vi "svfa_Check Data Valid [Dual FFT].vi"(0 "stimulus [X]":waveform(dbl)={"t0"=timestamp(0 s since 1904-01-01), "dt"=1.953125e-05, "Y"=[]}, 1 "response [Y]":waveform(dbl)={"t0"=timestamp(0 s since 1904-01-01), "dt"=1.953125e-05, "Y"=[]}, 2 "window":T3=1 items=["None"=0, "Hanning"=1, "Hamming"=2, "Blackman-Harris"=3, "Exact Blackman"=4, "Blackman"=5, "Flat Top"=6, "4 Term B-Harris "=7, "7 Term B-Harris"=8, "Low Sidelobe"=9, "Force - Exponential"=10, "Blackman Nuttall"=11, "Triangle"=30, "Bartlett-Hanning"=31, "Bohman"=32, "Parzen"=33, "Welch"=34, "Kaiser"=60, "Dolph-Chebyshev"=61, "Gaussian"=62], 3 "force/exp settings":T2={"force window [%]"=50.0, "exp window [%]"=10.0} {"exp window [%]" min=0.0 max=100.0 format="%.2f"; "force window [%]" min=0.0 max=100.0 format="%.2f"}, 4 "averaging parameters":T5={"averaging mode"=enum."No averaging", "weighting mode"=enum."Linear", "number of averages"=10, "linear mode"=enum."Auto restart"}, 5 "error in (no error)":errorcluster, 7 "processing control in":T4(ring), 8 "restart averaging (F)":bool, 9 "FRF mode":enum16{"H1", "H2", "H3"}(ring), 10 "measurement":T1(ring)=enum."Frequency response") -> (11 "dup FRF mode":enum16{"H1", "H2", "H3"}(ring), 13 "processing control out":T4(ring), 14 "dup stimulus [X]":waveform(dbl)={"t0"=timestamp(0 s since 1904-01-01), "dt"=1.953125e-05, "Y"=[]}, 15 "dup response [Y]":waveform(dbl)={"t0"=timestamp(0 s since 1904-01-01), "dt"=1.953125e-05, "Y"=[]}, 16 "window":T3=1 items=["None"=0, "Hanning"=1, "Hamming"=2, "Blackman-Harris"=3, "Exact Blackman"=4, "Blackman"=5, "Flat Top"=6, "4 Term B-Harris "=7, "7 Term B-Harris"=8, "Low Sidelobe"=9, "Force - Exponential"=10, "Blackman Nuttall"=11, "Triangle"=30, "Bartlett-Hanning"=31, "Bohman"=32, "Parzen"=33, "Welch"=34, "Kaiser"=60, "Dolph-Chebyshev"=61, "Gaussian"=62], 17 "dup force/exp settings":T2={"force window [%]"=50.0, "exp window [%]"=10.0} {"exp window [%]" min=0.0 max=100.0 format="%.2f"; "force window [%]" min=0.0 max=100.0 format="%.2f"}, 18 "dup averaging parameters":T5={"averaging mode"=enum."No averaging", "weighting mode"=enum."Linear", "number of averages"=10, "linear mode"=enum."Auto restart"}, 19 "error out":errorcluster)   [LabVIEW 2017]
uses:
  <vilib>/addons/_NISVFA/_Shared subVIs/Controls/svc_Window [Dual FFT].ctl
  <vilib>/addons/_NISVFA/_Shared subVIs/Common/svc_Check for Waveform Parameter Continuity (1 Ch).vi
  <vilib>/addons/_NISVFA/_Shared subVIs/Common/svc_Check for Waveform Parameter Continuity (no state).vi
  <vilib>/addons/_NISVFA/_Shared subVIs/Common/svc_Get SV Channel Info.vi
  <vilib>/addons/_NISVFA/_Shared subVIs/Common/svc_Check dt for Equal Sample Rates.vi
  <vilib>/addons/_NISVFA/_Shared subVIs/Common/svc_Engineering Units to Unit Label.vi
  <vilib>/addons/_NISVFA/_Shared subVIs/Common/svc_Unit Label to Engineering Units.vi
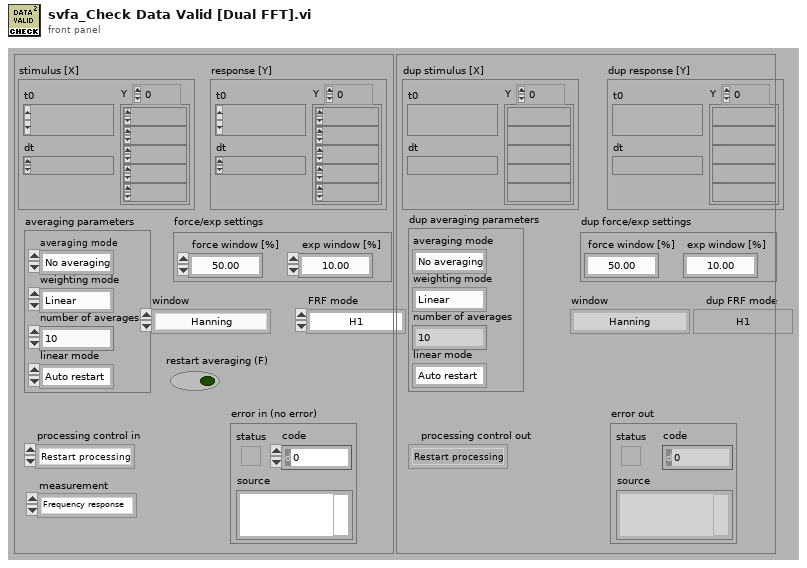
[diagram p1: front panel]
types:
  T1 = enum16{"Cross spectrum", "Frequency response", "Coherent output power"}
  T2 = cluster{"force window [%]":dbl, "exp window [%]":dbl}
  T3 = typedef "svc_Window [Dual FFT].ctl" = u32
  T4 = enum16{"Restart processing", "Continue processing", "Skip processing"}
  T5 = cluster{"averaging mode":enum16{"No averaging", "Vector averaging", "RMS averaging", "Peak hold"}, "weighting mode":enum16{"Linear", "Exponential"}, "number of averages":u32, "linear mode":enum16{"One shot", "Auto restart"}}
  T6 = cluster{"dt":bool, "t0 continuity":bool, "array length":bool, "channel info":bool, "name":bool}
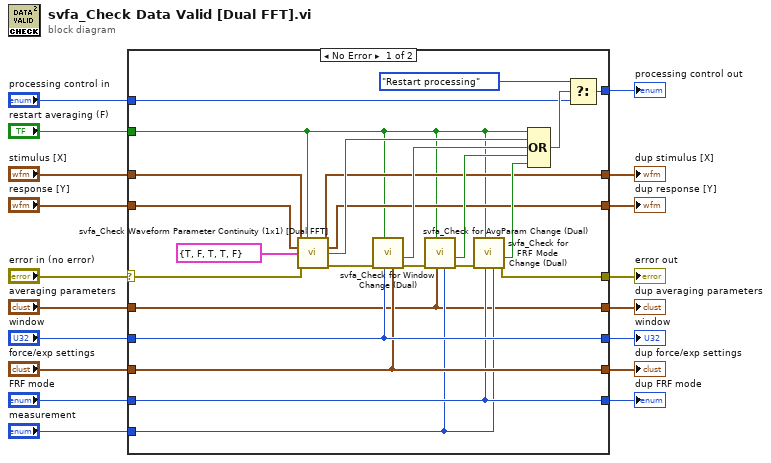
[diagram p0: block diagram]
diagram:
  n1 = case shown="No Error" "error in (no error)" {
    selector: "error in (no error)" -> [w22 w50]
    tunnel: [w20 w50] -> w18
    tunnel: "stimulus [X]" -> [w24 w44]
    tunnel: "response [Y]" -> [w27 w43]
    tunnel: "restart averaging (F)" -> [w21 _]
    tunnel: "processing control in" -> [w37 w47]
    tunnel: "FRF mode" -> [w39 w49]
    tunnel: "averaging parameters" -> [w19 w46]
    tunnel: "window" -> [w41 w45]
    tunnel: "force/exp settings" -> [w40 w48]
    tunnel: [w39 w49] -> w10
    tunnel: [w40 w48] -> w9
    tunnel: [w36 w47] -> w8
    tunnel: [w19 w46] -> w7
    tunnel: [w41 w45] -> w6
    tunnel: "measurement" -> [w33 _]
    tunnel: [w25 w44] -> w2
    tunnel: [w26 w43] -> w1
    frame No Error {
      n2 = call <vilib>:"svfa_Check Waveform Parameter Continuity (1x1) [Dual FFT].vi"("stimulus signal X [EUx]"=w24, "restart averaging (F)"=w21, "response signal Y [EUy]"=w27, "checks for channel parameter change"=T6 {"dt"=TRUE, "t0 continuity"=FALSE, "array length"=TRUE, "channel info"=TRUE, "name"=FALSE}, "error in"=w22) -> ("stimulus signal X [EUx]"=w25:waveform(dbl), "response signal Y [EUy]"=w26:waveform(dbl), "waveform parameter changed"=w28:bool, "error out"=w31:errorcluster)  [unwired: 5 in, 2 out]
      n3 = call <vilib>:"svfa_Check for Window Change (Dual).vi"("force/exp settings"=w40, "window"=w41, "restart averaging (F)"=w21, "error in (no error)"=w31) -> ("error out"=w35:errorcluster, "parameter has changed"=w29:bool)  [unwired: 6 in]
      n4 = call <vilib>:"svfa_Check for AvgParam Change (Dual).vi"("measurement"=w33, "averaging parameters"=w19, "restart averaging (F)"=w21, "error in (no error)"=w35) -> ("error out"=w32:errorcluster, "parameter has changed"=w30:bool)  [unwired: 6 in]
      n5 = call <vilib>:"svfa_Check for FRF Mode Change (Dual).vi"("measurement"=w33, "FRF mode"=w39, "restart"=w21, "error in (no error)"=w32) -> ("error out"=w20:errorcluster, "parameter has changed"=w34:bool)  [unwired: 6 in]
      n6 = Compound Arithmetic op=OR(w21, w28, w29, w30, w34) -> (w38:bool)
      n7 = Select(t=T4."Restart processing", s=w38, f=w37) -> (s? t:f=w36:T4)
    }
    frame Error {
    }
  }
  "dup stimulus [X]" <- w2
  "error out" <- w18
  "dup response [Y]" <- w1
  "dup averaging parameters" <- w7
  "processing control out" <- w8
  "window" <- w6
  "dup force/exp settings" <- w9
  "dup FRF mode" <- w10
